vi "Read Counter.vi"(4 "TL Calling Location":string, 6 "error In":errorcluster, 9 "TASK ID":u32) -> (0 "error out":errorcluster, 1 "counter overflow?":bool, 2 "time (secs)":sgl format="%.8f", 3 "count":u32)   [LabVIEW 2012]
doc: "DESCRIPTION:\nThis VI counts rising edges, using an NI-TIO based device (e.g.: 6602). The counter increments its event count everytime a pulse comes into its source input. The counters only increments between the rising edge of the aux line and the rising edge of the gate. The current value of the counter is read when the counter is finished or an error occurs. \n\n\n\nINSTRUCTIONS:\n1. Enter the device and counter you want use.\n2. Optional controls are located on the left side of the front panel. You will have to use your scroll bar to reach these. \n3. Connect your signals as described below in I/O CONNECTIONS.\n4. Run the VI.\n\n\nKEY PARAMETERS:\nCounter Group Config.vi: task type = two edge separation measurement\nCounter Source (NI-TIO).vi: Source Specification\nCounter Gate (NI-TIO).vi: Gate Specification\nCounter Aux Line (NI-TIO): Aux Line Specification\nCounter Get Attribute.vi: armed, TC Reached, count\nCounter Control.vi: Program, Reset\n\n\n\nI/O CONNECTIONS:\nConnect the start signal to the aux line input of the selected counter. Connect the stop signal to the gate input of the selected counter. \nIf you selected the Source Selection to be \"PFI line\", connect your event count base signal to the PFI line indicated by \"Source PFI line number used\". (If you selected \"Internal Timebase\", no source connection is necessary.)\n\nNOTE: For actual I/O pin numbers, please refer to your hardware user manual.\n\n\n\nDAQ VIs USED:\nCounter Group Config.vi\nCounter Source (NI-TIO).vi\nCounter Gate (NI-TIO).vi\nCounter Aux Line (NI-TIO)\nCounter Get Attribute.vi\nCounter Control.vi"
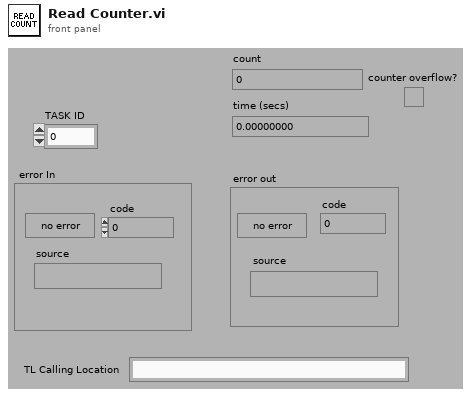
[diagram p1: front panel]
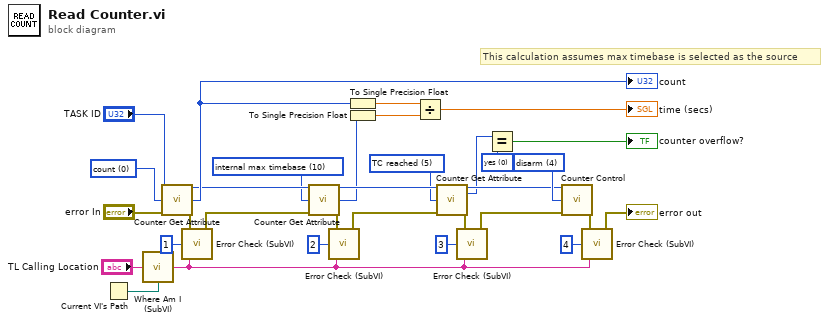
[diagram p0: block diagram]
diagram:
  w22 = u32 0 items=["yes", "no", "high", "low"] ("attribute value type")
  w23 = u32 5 items=["count", "saved count", "count available", "available points", "armed", "TC reached", "done", "output state", "read mark", "write mark", "internal max timebase", "max prescale", "read mark high snapshot", "read mark low snapshot", "write mark high snapshot", "write mark low snapshot", "backlog high snapshot", "backlog low snapshot", "armed snapshot"] ("attribute ID")
  w24 = u32 10 items=["count", "saved count", "count available", "available points", "armed", "TC reached", "done", "output state", "read mark", "write mark", "internal max timebase", "max prescale", "read mark high snapshot", "read mark low snapshot", "write mark high snapshot", "write mark low snapshot", "backlog high snapshot", "backlog low snapshot", "armed snapshot"] ("attribute ID")
  w25 = u32 0 items=["count", "saved count", "count available", "available points", "armed", "TC reached", "done", "output state", "read mark", "write mark", "internal max timebase", "max prescale", "read mark high snapshot", "read mark low snapshot", "write mark high snapshot", "write mark low snapshot", "backlog high snapshot", "backlog low snapshot", "armed snapshot"] ("attribute ID")
  w32 = u32 4 items=["program", "reset", "arm", "prepare", "disarm", "count up", "count down", "switch cycle", "snapshot"] ("control code")
  # "This calculation assumes max timebase is selected as the source"
  n1 = Current VI's Path() -> (path=w3:path)
  n2 = call "Where Am I (SubVI).vi"("TL Calling Location"="TL Calling Location", "Call VI path"=w3) -> ("I'm here"=w1:string)
  n3 = call "Counter Get Attribute.vi"("task ID"="TASK ID", "attribute ID"=w25, "error in (no error)"="error In") -> ("task ID out"=w30:u32, "attribute value number"=w31:u32, "error out"=w14:errorcluster)  [unwired: 9 in, 1 out]
  "count" <- w31
  n4 = call "Error Check (SubVI).vi"("calling VI"=w1, "tag #"=1 ("code locator tag #"), "error IN"=w14) -> ("error OUT"=w13:errorcluster)  [unwired: 2 in]
  n5 = call "Counter Get Attribute.vi"("task ID"=w30, "attribute ID"=w24, "error in (no error)"=w13) -> ("task ID out"=w29:u32, "attribute value number"=w18:u32, "error out"=w8:errorcluster)  [unwired: 9 in, 1 out]
  n6 = call "Error Check (SubVI).vi"("calling VI"=w1, "tag #"=2 ("code locator tag #"), "error IN"=w8) -> ("error OUT"=w7:errorcluster)  [unwired: 2 in]
  n7 = To Single Precision Float(number=w31) -> (single precision float=w17:sgl)
  n8 = To Single Precision Float(number=w18) -> (single precision float=w16:sgl)
  n9 = Divide(x=w17, y=w16) -> (x/y=→"time (secs)":sgl)
  n10 = call "Counter Get Attribute.vi"("task ID"=w29, "attribute ID"=w23, "error in (no error)"=w7) -> ("task ID out"=w28:u32, "attribute value type"=w21:u32, "error out"=w6:errorcluster)  [unwired: 9 in, 1 out]
  n11 = call "Error Check (SubVI).vi"("calling VI"=w1, "tag #"=3 ("code locator tag #"), "error IN"=w6) -> ("error OUT"=w5:errorcluster)  [unwired: 2 in]
  n12 = Equal?(x=w21, y=w22) -> (x = y?=→"counter overflow?":bool)
  n13 = call "Counter Control.vi"("task ID"=w28, "control code"=w32, "error in (no error)"=w5) -> ("error out"=w9:errorcluster)  [unwired: 11 in, 1 out]
  n14 = call "Error Check (SubVI).vi"("calling VI"=w1, "tag #"=4 ("code locator tag #"), "error IN"=w9) -> ("error OUT"=→"error out":errorcluster)  [unwired: 2 in]
